vi "test4-SyncMessageWithError_API.vi"(8 "error in":errorcluster, 11 "TestCase in":refnum<class "testcase-CSMMessage.lvclass">) -> (0 "error out":errorcluster, 3 "TestCase out":refnum<class "testcase-CSMMessage.lvclass">)   [LabVIEW 2017, in "testcase-CSMMessage.lvclass"]
uses:
  testcase-CSMMessage.lvclass
  82a3f3a0-c761-4c70-9aec-dba3e6f930bc.vi
  src/user.lib/_NEVSTOP/Communicable State Machine(CSM)/AdvanceAPI/CSM - Make String Arguments Safe.vi
  src/user.lib/_NEVSTOP/Communicable State Machine(CSM)/AdvanceAPI/CSM - Keywords.vi
  <vilib>/addons/_JKI Toolkits/VI Tester/TestCase.llb/TestCase.lvclass
  src/user.lib/_NEVSTOP/Communicable State Machine(CSM)/Communicable State Machine.lvlib
  C:/Program Files (x86)/National Instruments/LabVIEW 2017/vi.lib/addons/_JKI Toolkits/VI Tester/TestCase.llb/TestCase.lvclass
panel:
  out "LoopCount":i32
  out "concatenated string":string
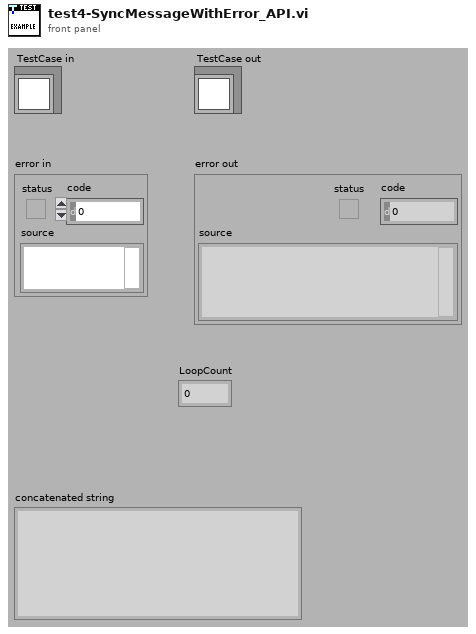
[diagram p1: front panel]
types:
  T1 = cluster{"Arguments":string, "Response":string, "error":errorcluster}
  T2 = cluster{"status":bool, "code":bool, "source":bool}
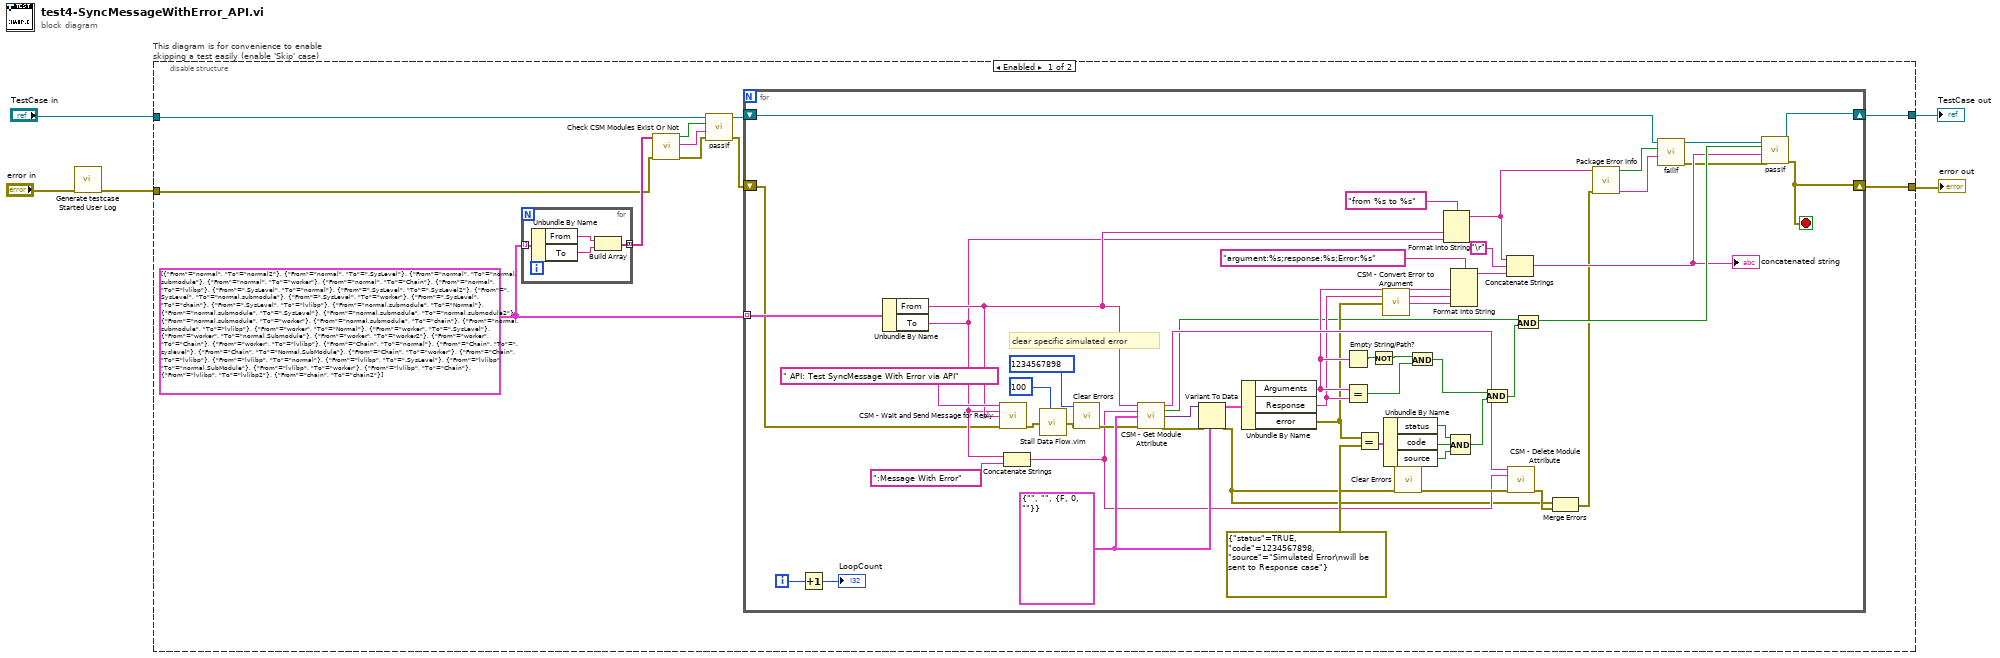
[diagram p0: block diagram]
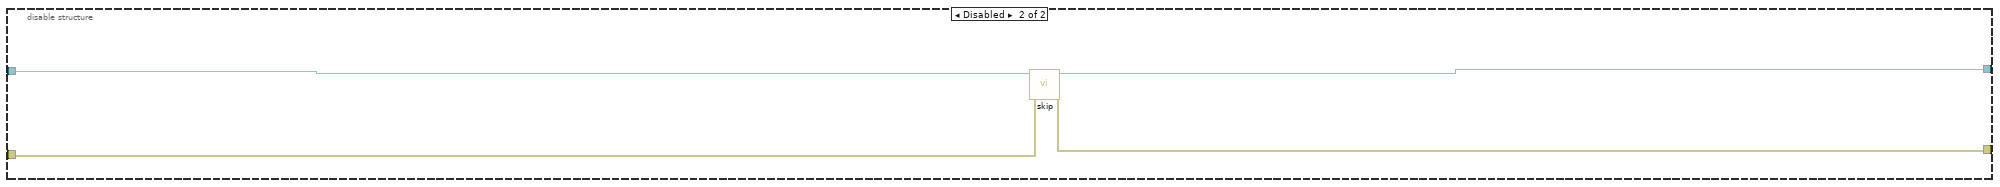
[diagram p2: hidden frame]
diagram:
  n1 = call "Generate testcase Started User Log.vi"("Error In"="error in") -> ("error out"=w1:errorcluster)  [unwired: 10 in]
  n2 = disable-structure "This diagram is for convenience to enable skipping a test easily (enable 'Skip' case)" shown="Enabled" {
    disable-tunnel: "TestCase in" -> [w9 w77]
    disable-tunnel: [w7 w75] -> w2
    disable-tunnel: [w6 w76] -> w4
    disable-tunnel: w1 -> [w10 w74]
    frame Enabled {
      w12 = cluster{"From":string, "To":string}[] [{"From"="normal", "To"="normal2"}, {"From"="normal", "To"=".SysLevel"}, {"From"="normal", "To"="normal.submodule"}, {"From"="normal", "To"="worker"}, {"From"="normal", "To"="Chain"}, {"From"="normal", "To"="lvlibp"}, {"From"=".SysLevel", "To"="normal"}, {"From"=".SysLevel", "To"=".SysLevel2"}, {"From"=".SysLevel", "To"="normal.submodule"}, {"From"=".SysLevel", "To"="worker"}, {"From"=".SysLevel", "To"="chain"}, {"From"=".SysLevel", "To"="lvlibp"}, {"From"="normal.submodule", "To"="Normal"}, {"From"="normal.submodule", "To"=".SysLevel"}, {"From"="normal.submodule", "To"="normal.submodule2"}, {"From"="normal.submodule", "To"="worker"}, {"From"="normal.submodule", "To"="chain"}, {"From"="normal.submodule", "To"="lvlibp"}, {"From"="worker", "To"="Normal"}, {"From"="worker", "To"=".SysLevel"}, {"From"="worker", "To"="normal.Submodule"}, {"From"="worker", "To"="worker2"}, {"From"="worker", "To"="Chain"}, {"From"="worker", "To"="lvlibp"}, {"From"="Chain", "To"="normal"}, {"From"="Chain", "To"=".syslevel"}, {"From"="Chain", "To"="Normal.SubModule"}, {"From"="Chain", "To"="worker"}, {"From"="Chain", "To"="lvlibp"}, {"From"="lvlibp", "To"="normal"}, {"From"="lvlibp", "To"=".SysLevel"}, {"From"="lvlibp", "To"="normal.SubModule"}, {"From"="lvlibp", "To"="worker"}, {"From"="lvlibp", "To"="Chain"}, {"From"="lvlibp", "To"="lvlibp2"}, {"From"="chain", "To"="chain2"}]
      n3 = for {
        tunnel: w12 -> [w20] mode=indexing
        tunnel: [w17] -> w15 mode=concatenating
        n4 = Unbundle By Name(w20) -> ("From"=w19:string, "To"=w18:string)
        n5 = Build Array(w19, w18) -> (w17:string[])
      }
      n6 = call "Check CSM Modules Exist Or Not.vi"("error in"=w10, "CSM names in"=w15) -> ("error out"=w13:errorcluster, "Debug string"=w14:string, "All Modules Exist?"=w16:bool)  [unwired: 7 in]
      n7 = call-dynamic "passIf.vi"("error in (no error)"=w13, "message (\"\")"=w14, "pass"=w16, "TestCase in"=w9) -> ("error out"=w11:errorcluster, "TestCase out"=w8:refnum<class "testcase-CSMMessage.lvclass">)  [unwired: 6 in]
      n8 = for {
        tunnel: w12 -> [w66] mode=indexing
        shift-right: [w73] -> w7
        shift-left: w8 -> [w25]
        shift-right: [w52] -> w6
        shift-left: w11 -> [w31]
        i -> [w34]
        stop <- w52 stop-if-true
        w70 = T1 {"Arguments"="", "Response"="", "error"={"status"=FALSE, "code"=0, "source"=""}}
        # "clear specific simulated error"
        n9 = Increment(x=w34) -> (x+1=→"LoopCount":i32)
        n10 = Unbundle By Name(w66) -> ("From"=w43:string, "To"=w41:string)
        n11 = call "CSM - Wait and Send Message for Reply.vi"("State"=" API: Test SyncMessage With Error via API", "Arguments (\"\")"=w41, "Target Module"=w43, "Error In (No Error)"=w31) -> ("error out"=w39:errorcluster)  [unwired: 8 in, 3 out]
        n12 = Concatenate Strings(w41, ":Message With Error" ("State")) -> (w40:string)
        n13 = call "Stall Data Flow.vim"("value in"=w39, "milliseconds to wait"=u32 100) -> ("value out"=w38:errorcluster)  [unwired: 1 out]
        n14 = call <vilib>:"Clear Errors.vi"("error in (no error)"=w38, "specific error code to clear (0: all)"=1234567898) -> ("error out"=w44:errorcluster)  [unwired: 4 in, 1 out]
        n15 = call "CSM - Get Module Attribute.vi"("CSM Name"=w43, "Attribute"=w40, "Default Value (Empty Variant)"=w70, "Error In"=w44) -> ("CSM Name (Dup)"=w64:string, "Found"=w36:bool, "Value"=w35:variant, "error out"=w71:errorcluster)  [unwired: 7 in, 1 out]
        n16 = Variant To Data(error in=w71, type=w70, Variant=w35) -> (data=w69:T1, error out=w29:errorcluster)
        n17 = Unbundle By Name(w69) -> ("Arguments"=w59:string, "Response"=w58:string, "error"=w51:errorcluster)
        n18 = Empty String/Path?(string/path=w59) -> (empty?=w63:bool)
        n19 = Equal?(x=w59, y=w58) -> (x = y?=w61:bool)
        n20 = Equal?(x=w51, y=errorcluster {"status"=TRUE, "code"=1234567898, "source"="Simulated Error\nwill be sent to Response case"} ("error out")) -> (x = y?=w49:T2)
        n21 = Not(x=w63) -> (.not. x?=w62:bool)
        n22 = call "CSM - Convert Error to Argument.vi"("Error"=w51) -> ("Argument"=w57:string)  [unwired: 4 in]
        n23 = Unbundle By Name(w49) -> ("status"=w48:bool, "code"=w47:bool, "source"=w46:bool)
        n24 = call <vilib>:"Clear Errors.vi"("error in (no error)"=w29) -> ("error out"=w53:errorcluster)  [unwired: 5 in, 1 out]
        n25 = And(x=w62, y=w61) -> (x .and. y?=w60:bool)
        n26 = Format Into String(format string="from %s to %s", w43, w41) -> (resulting string=w21:string)  [unwired: 2 in, 1 out]
        n27 = Format Into String(format string="argument:%s;response:%s;Error:%s", w59, w58, w57) -> (resulting string=w56:string)  [unwired: 2 in, 1 out]
        n28 = Compound Arithmetic op=AND(w48, w47, w46) -> (w45:bool)
        n29 = And(x=w60, y=w45) -> (x .and. y?=w68:bool)
        n30 = Concatenate Strings(w21, "\r", w56) -> (w28:string)
        "concatenated string" <- w28
        n31 = call "CSM - Delete Module Attribute.vi"("CSM Name"=w64, "Attribute"=w40, "Error In"=w53) -> ("error out"=w30:errorcluster)  [unwired: 9 in, 3 out]
        n32 = And(x=w36, y=w68) -> (x .and. y?=w67:bool)
        n33 = Merge Errors(w29, w30) -> (w22:errorcluster)
        n34 = call "Package Error Info.vi"("error in"=w22, "String in"=w21) -> ("packed error info out"=w26:string, "error status"=w27:bool)  [unwired: 8 in]
        n35 = call-dynamic "failIf.vi"("message (\"\")"=w26, "fail"=w27, "TestCase in"=w25) -> ("error out"=w23:errorcluster, "TestCase out"=w24:refnum<class "testcase-CSMMessage.lvclass">)  [unwired: 7 in]
        n36 = call-dynamic "passIf.vi"("error in (no error)"=w23, "message (\"\")"=w28, "pass"=w67, "TestCase in"=w24) -> ("error out"=w52:errorcluster, "TestCase out"=w73:refnum<class "testcase-CSMMessage.lvclass">)  [unwired: 6 in]
      }
    }
    frame Disabled {
      # "skip test result while test is under development"
      n37 = call <vilib>:"skip.vi"("error in (no error)"=w74, "TestCase in"=w77) -> ("error out"=w76:errorcluster, "TestCase out"=w75:refnum<class "testcase-CSMMessage.lvclass">)  [unwired: 8 in]
    }
  }
  "error out" <- w4
  "TestCase out" <- w2
